vi "Obtain Request Events.vi"(8 "error in":errorcluster, 10 "Create New? (F)":bool) -> (0 "error out":errorcluster, 2 "Manejador archivo Request Events":T1)   [LabVIEW 2020, in "Manejador archivo.lvlib"]
doc: "This VI Obtains/Creates the Requests events that will be used for other modules to communicate with the module that owns this VI. These Requests events will be accessed only via Public API methods for this module.\n\n<b>NOTE</b>: The contents of this VI are automatically generated and modified by the <b>Tools > DQMH Consortium > DQMH</b> utilities. Consider using those utilities instead of making your own modifications to this VI.\n_____\nBased on DQMH Dev Tools: Project Template 7.1.0.1490."
uses:
  Manejador archivo.lvlib
  Request Events--cluster.ctl
  Stop Argument--cluster.ctl
  Show Panel Argument--cluster.ctl
  Hide Panel Argument--cluster.ctl
  Get Module Execution Status Argument--cluster.ctl
  Show Diagram Argument--cluster.ctl
  Set Column Headers Argument--cluster.ctl
  View File Argument--cluster.ctl
  Set File Path Argument--cluster.ctl
  Set File Settings Argument--cluster.ctl
  Log Data Argument--cluster.ctl
  Log Data (Reply Payload)--cluster.ctl
  Set File Format Argument--cluster.ctl
  File Formats--enum.ctl
  Close File Argument--cluster.ctl
  Get Number of Columns Argument--cluster.ctl
  Get Number of Columns (Reply Payload)--cluster.ctl
panel:
  # "NOTE: The contents of this VI are automatically generated and modified by the Tools > DQMH Consortium > DQMH utilities. Consider using those utilities instead of making your own modifications to this VI."
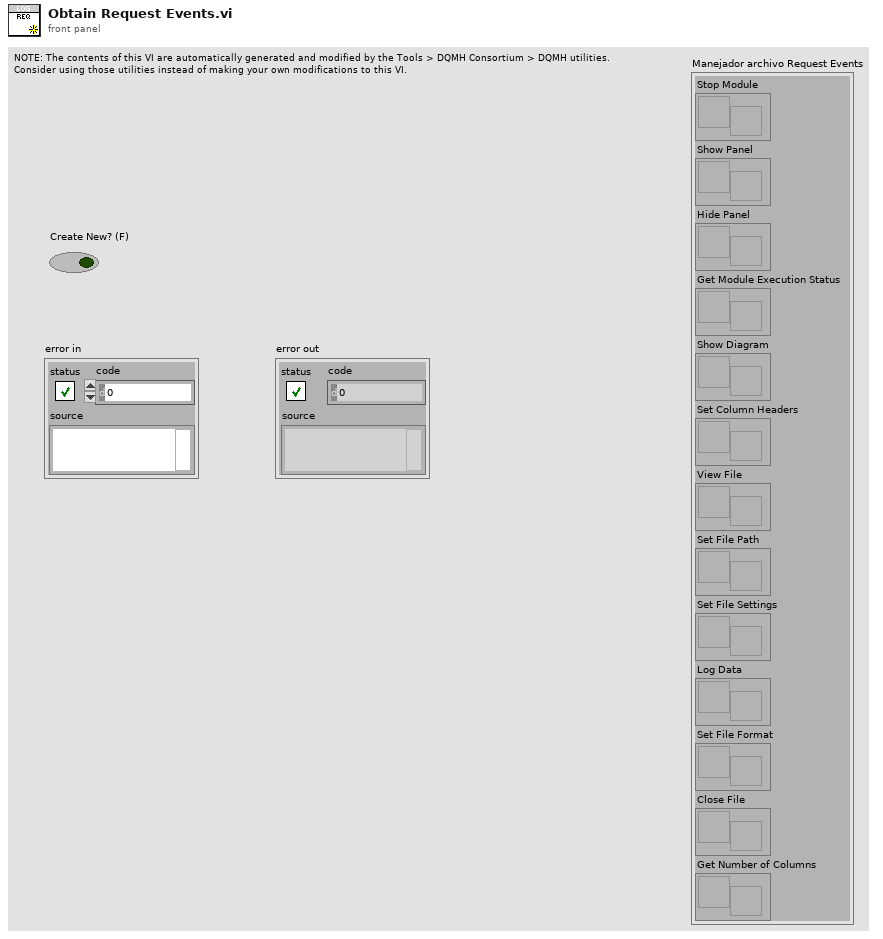
[diagram p1: front panel]
types:
  T1 = typedef "Manejador archivo.lvlib/Request Events--cluster.ctl" = cluster{"Stop Module":refnum<user-event>, "Show Panel":refnum<user-event>, "Hide Panel":refnum<user-event>, "Get Module Execution Status":refnum<user-event>, "Show Diagram":refnum<user-event>, "Set Column Headers":refnum<user-event>, "View File":refnum<user-event>, "Set File Path":refnum<user-event>, "Set File Settings":refnum<user-event>, "Log Data":refnum<user-event>, "Set File Format":refnum<user-event>, "Close File":refnum<user-event>, "Get Number of Columns":refnum<user-event>}
  T2 = typedef "Manejador archivo.lvlib/Get Number of Columns Argument--cluster.ctl" = cluster{"Wait Notifier":refnum<notifier>, "wait for reply":bool}
  T3 = typedef "Manejador archivo.lvlib/Close File Argument--cluster.ctl" = cluster{"Boolean":bool}
  T4 = typedef "Manejador archivo.lvlib/Set File Format Argument--cluster.ctl" = cluster{"Format":T5}
  T5 = typedef "Manejador archivo.lvlib/File Formats--enum.ctl" = enum16{"TDMS", "CSV"}
  T6 = typedef "Manejador archivo.lvlib/Log Data Argument--cluster.ctl" = cluster{"Data":dbl[], "Wait Notifier":refnum<notifier>, "wait for reply":bool}
  T7 = typedef "Manejador archivo.lvlib/Set File Settings Argument--cluster.ctl" = cluster{"Save Time Stamp":bool, "Delimiter":enum16{"Tab", "Coma"}}
  T8 = typedef "Manejador archivo.lvlib/Set File Path Argument--cluster.ctl" = cluster{"Path":path}
  T9 = typedef "Manejador archivo.lvlib/View File Argument--cluster.ctl" = cluster{"Boolean":bool}
  T10 = typedef "Manejador archivo.lvlib/Set Column Headers Argument--cluster.ctl" = cluster{"Headers":string[]}
  T11 = typedef "Manejador archivo.lvlib/Hide Panel Argument--cluster.ctl" = cluster{"Hide Panel?":bool}
  T12 = typedef "Manejador archivo.lvlib/Show Panel Argument--cluster.ctl" = cluster{"Show Panel?":bool}
  T13 = typedef "Manejador archivo.lvlib/Show Diagram Argument--cluster.ctl" = cluster{"Debug?":bool}
  T14 = typedef "Manejador archivo.lvlib/Get Module Execution Status Argument--cluster.ctl" = cluster{"Running?":bool}
  T15 = typedef "Manejador archivo.lvlib/Stop Argument--cluster.ctl" = cluster{"Origin":string, "Exit via Stop Module Req?":bool, "Wait for Module to stop?":bool}
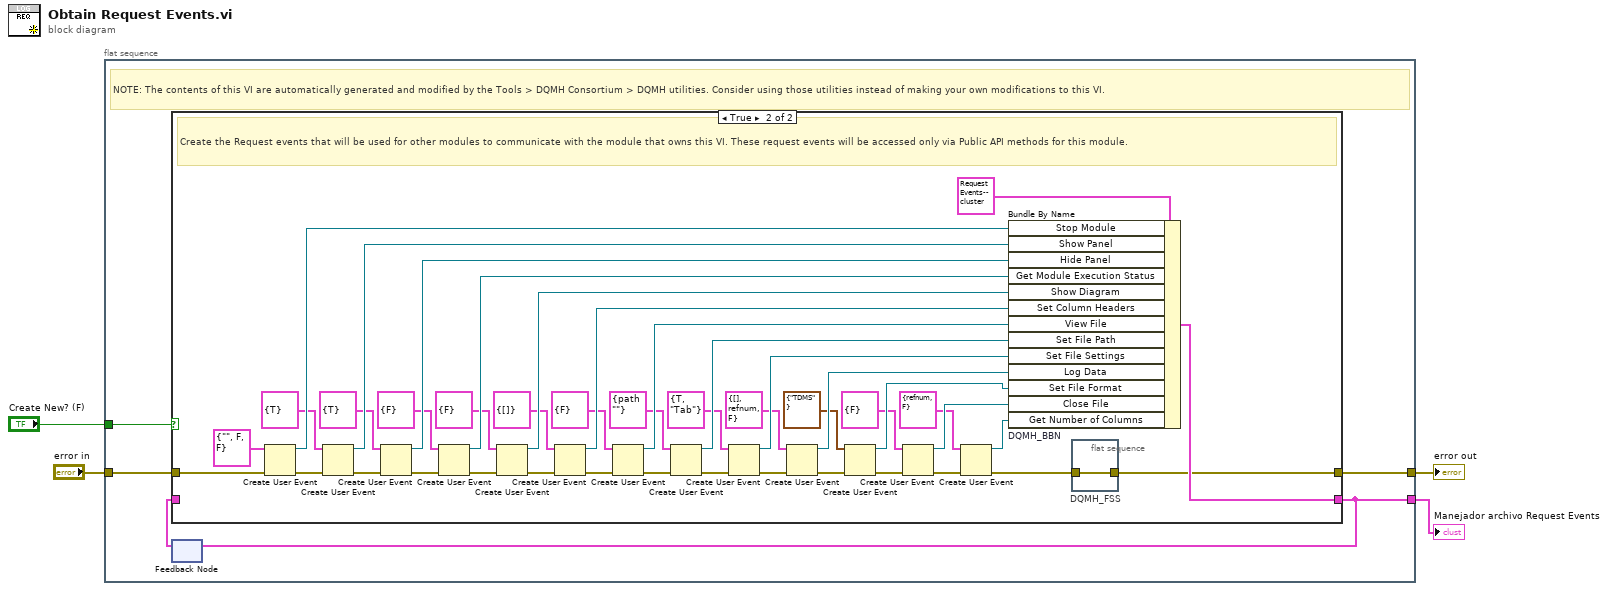
[diagram p0: block diagram]
diagram:
  n1 = flat-sequence {
    tunnel: [w9] -> w4
    tunnel: "error in" -> [w8]
    tunnel: [w6] -> w2
    tunnel: "Create New? (F)" -> [w5]
    frame #0 {
      # "NOTE: The contents of this VI are automatically generated and modified by the Tools > DQMH Consortium > DQMH utilities. Consider using those utilities instead of making your own modifications to this VI."
      n2 = feedback #1() -> (w7:T1)  [unwired: 1 in]
      n3 = case shown="True" w5 {
        tunnel: [w10 w44] -> w9
        tunnel: w8 -> [w10 w54]
        tunnel: [w11 w51] -> w6
        tunnel: w7 -> [w11 _]
        frame False {
          # "Obtain the Request events that were created in a previous call to this VI."
        }
        frame True {
          # "Create the Request events that will be used for other modules to communicate with the module that owns this VI. These request events will be accessed only via Public API methods for this module."
          n4 = Create User Event(user event datatype=T15 {"Origin"="", "Exit via Stop Module Req?"=FALSE, "Wait for Module to stop?"=FALSE} ("Stop Argument"), error in=w54) -> (user event=w52:refnum<user-event>, error out=w49:errorcluster)
          n5 = Create User Event(user event datatype=T12 {"Show Panel?"=TRUE} ("Show Panel Argument"), error in=w49) -> (user event=w48:refnum<user-event>, error out=w47:errorcluster)
          n6 = Create User Event(user event datatype=T11 {"Hide Panel?"=TRUE} ("Hide Panel Argument"), error in=w47) -> (user event=w46:refnum<user-event>, error out=w45:errorcluster)
          n7 = Create User Event(user event datatype=T14 {"Running?"=FALSE} ("Get Module Execution Status Argument"), error in=w45) -> (user event=w42:refnum<user-event>, error out=w43:errorcluster)
          n8 = Create User Event(user event datatype=T13 {"Debug?"=FALSE} ("Show Diagram Argument"), error in=w43) -> (user event=w39:refnum<user-event>, error out=w40:errorcluster)
          n9 = Create User Event(user event datatype=T10 {"Headers"=[]} ("Set Column Headers Argument"), error in=w40) -> (user event=w34:refnum<user-event>, error out=w35:errorcluster)
          n10 = Create User Event(user event datatype=T9 {"Boolean"=FALSE} ("View File Argument"), error in=w35) -> (user event=w31:refnum<user-event>, error out=w32:errorcluster)
          n11 = Create User Event(user event datatype=T8 {"Path"=path ""} ("Set File Path Argument"), error in=w32) -> (user event=w28:refnum<user-event>, error out=w29:errorcluster)
          n12 = Create User Event(user event datatype=T7 {"Save Time Stamp"=TRUE, "Delimiter"=enum."Tab"} ("Set File Settings Argument"), error in=w29) -> (user event=w25:refnum<user-event>, error out=w26:errorcluster)
          n13 = Create User Event(user event datatype=T6 {"Data"=[], "Wait Notifier"=refnum, "wait for reply"=FALSE} ("Log Data Argument"), error in=w26) -> (user event=w22:refnum<user-event>, error out=w23:errorcluster)
          n14 = Create User Event(user event datatype=T4 {"Format"=enum."TDMS"} ("Set File Format Argument"), error in=w23) -> (user event=w19:refnum<user-event>, error out=w20:errorcluster)
          n15 = Create User Event(user event datatype=T3 {"Boolean"=FALSE} ("Close File Argument"), error in=w20) -> (user event=w16:refnum<user-event>, error out=w17:errorcluster)
          n16 = Create User Event(user event datatype=T2 {"Wait Notifier"=refnum, "wait for reply"=FALSE} ("Get Number of Columns Argument"), error in=w17) -> (user event=w13:refnum<user-event>, error out=w14:errorcluster)
          n17 = Bundle By Name "DQMH_BBN"(cluster=T1 {"Stop Module"=refnum, "Show Panel"=refnum, "Hide Panel"=refnum, "Get Module Execution Status"=refnum, "Show Diagram"=refnum, "Set Column Headers"=refnum, "View File"=refnum, "Set File Path"=refnum, "Set File Settings"=refnum, "Log Data"=refnum, "Set File Format"=refnum, "Close File"=refnum, "Get Number of Columns"=refnum} ("output cluster"), "Stop Module"=w52, "Show Panel"=w48, "Hide Panel"=w46, "Get Module Execution Status"=w42, "Show Diagram"=w39, "Set Column Headers"=w34, "View File"=w31, "Set File Path"=w28, "Set File Settings"=w25, "Log Data"=w22, "Set File Format"=w19, "Close File"=w16, "Get Number of Columns"=w13) -> (w51:T1)
          n18 = flat-sequence "DQMH_FSS" {
            tunnel: w14 -> [w55]
            tunnel: [w55] -> w44
            frame #0 {
            }
          }
        }
      }
      n19 = feedback-in #1(w6) -> ()
    }
  }
  "Manejador archivo Request Events" <- w2
  "error out" <- w4
